vi "LiDAR Avoid Obstacle.vi"(0 "Measurement Data":i32[](array[numeric]), 5 "Input Params":cluster{"angle":dbl[], "id":i32[], "kk":dbl[]}) -> (4 "Output data":T1, 6 "Obs_angle":dbl)   [LabVIEW 2016]
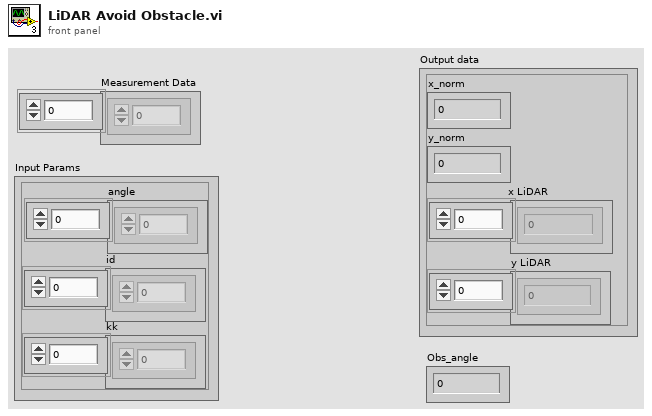
[diagram p1: front panel]
types:
  T1 = cluster{"x_norm":dbl, "y_norm":dbl, "x LiDAR":dbl[], "y LiDAR":dbl[]}
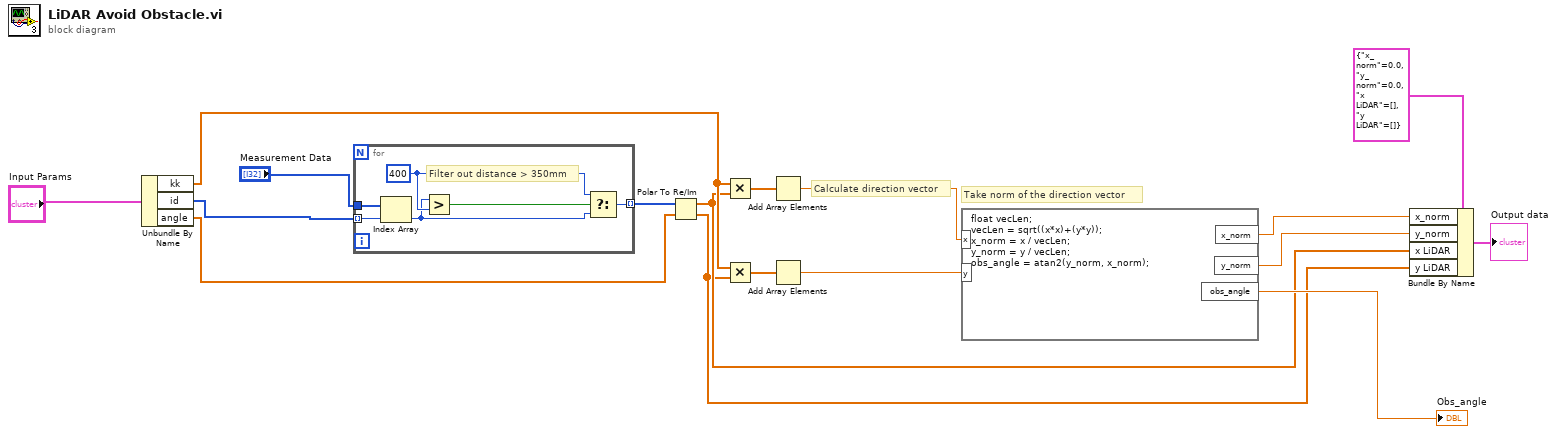
[diagram p0: block diagram]
diagram:
  # "Calculate direction vector"
  # "Take norm of the direction vector"
  n1 = Unbundle By Name("Input Params") -> ("kk"=w8:dbl[], "id"=w9:i32[], "angle"=w10:dbl[])
  n2 = for {
    tunnel: "Measurement Data" -> [w22]
    tunnel: w9 -> [w21] mode=indexing
    tunnel: [w18] -> w17 mode=indexing
    w23 = 400 ("y")
    # "Filter out distance > 350mm"
    n3 = Index Array(array=w22, index=w21) -> (element=w19:i32)
    n4 = Greater?(x=w19, y=w23) -> (0:w20:bool)
    n5 = Select(t=w23, s=w20, f=w19) -> (s? t:f=w18:i32)
  }
  n6 = Polar To Re/Im(2:w10, 3:w17) -> (0:w4:dbl[], 1:w5:dbl[])
  n7 = Multiply(x=w8, y=w5) -> (x*y=w13:dbl[])
  n8 = Multiply(x=w8, y=w4) -> (x*y=w14:dbl[])
  n9 = Add Array Elements(numeric array=w13) -> (sum=w12:dbl)
  n10 = Add Array Elements(numeric array=w14) -> (sum=w15:dbl)
  n11 = formula code="float vecLen;\nvecLen = sqrt((x*x)+(y*y));\nx_norm = x / vecLen;\ny_norm = y / vecLen;\nobs_angle = atan2(y_norm, x_norm);"("x"=w12, "y"=w15) -> ("y_norm"=w6:dbl, "x_norm"=w7:dbl, "obs_angle"=→"Obs_angle":dbl)
  n12 = Bundle By Name(cluster=T1 {"x_norm"=0.0, "y_norm"=0.0, "x LiDAR"=[], "y LiDAR"=[]} ("output cluster 2"), "x_norm"=w7, "y_norm"=w6, "x LiDAR"=w5, "y LiDAR"=w4) -> (→"Output data":T1)
